vi "Get Resolution.vi"(0 "Image":T1, 11 "error in (no error)":errorcluster) -> (4 "X Resolution":i32, 6 "Y Resolution":i32, 8 "Image Area:Size:All Elements":cluster{"Width":u32, "Height":u32}, 10 "valid Image":bool, 15 "error out":errorcluster)   [LabVIEW 2020]
uses:
  <vilib>/vision/Image Controls.llb/IMAQ Image.ctl
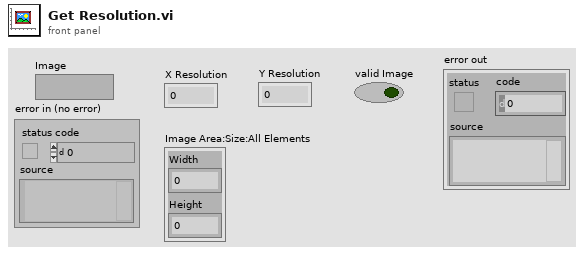
[diagram p1: front panel]
types:
  T1 = typedef "IMAQ Image.ctl" = refnum<image>
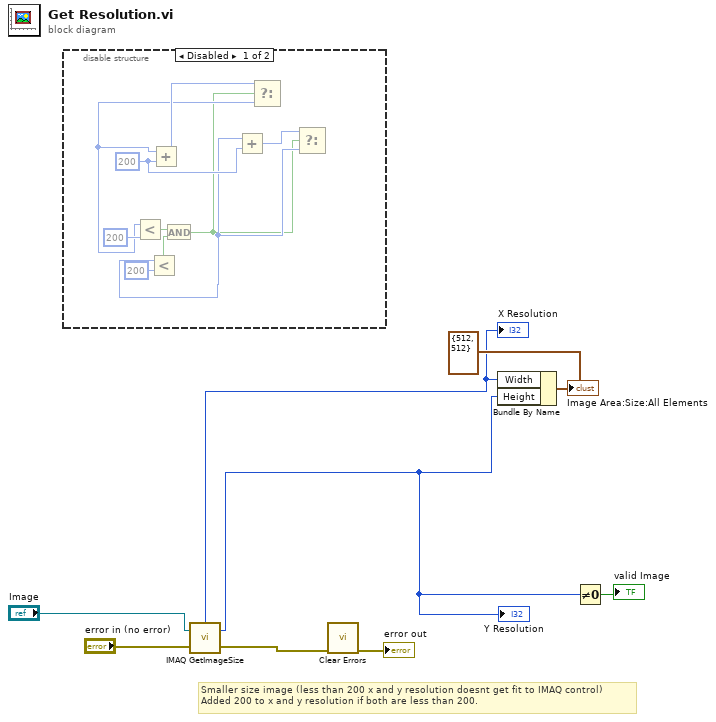
[diagram p0: block diagram]
diagram:
  # "Smaller size image (less than 200 x and y resolution doesnt get fit to IMAQ control)\nAdded 200 to x and y resolution if both are less than 200."
  n1 = disable-structure shown="Disabled" {
    frame Disabled {
      w20 = 200 ("y")
      n2 = Add(y=w20) -> (x=w14:i32, x+y=w15:i32)
      n3 = Less?(x=w14, y=200) -> (x < y?=w12:bool)
      n4 = Add(y=w20) -> (x=w16:i32, x+y=w17:i32)
      n5 = Less?(x=w16, y=200) -> (x < y?=w11:bool)
      n6 = And(x=w12, y=w11) -> (x .and. y?=w10:bool)
      n7 = Select(t=w15, s=w10, f=w14) -> (s? t:f=w13:i32)
      n8 = Select(t=w17, s=w10, f=w16) -> ()  [unwired: 1 out]
    }
    frame Enabled {
    }
  }
  n9 = call "IMAQ GetImageSize"("Image"="Image", "error in (no error)"="error in (no error)") -> ("Y Resolution"=w1:i32, "X Resolution"=w2:i32, "error out"=w8:errorcluster)  [unwired: 2 in]
  "Y Resolution" <- w1
  "X Resolution" <- w2
  n10 = call <vilib>:"Clear Errors.vi"("error in (no error)"=w8) -> ("error out"=→"error out":errorcluster)  [unwired: 5 in, 1 out]
  n11 = Bundle By Name(cluster=cluster{"Width":u32, "Height":u32} {"Width"=512, "Height"=512} ("Image Area:Size:All Elements"), "Width"=w2, "Height"=w1) -> (→"Image Area:Size:All Elements":cluster{"Width":u32, "Height":u32})
  n12 = Not Equal To 0?(x=w1) -> (x != 0?=→"valid Image":bool)
